vi "ConfigFiles.vi"   [LabVIEW 2016]
uses:
  <vilib>/Utility/config.llb/Read Key (String).vi
  Robot Global Data.vi
  <vilib>/Utility/config.llb/NI_LVConfig.lvlib
types:
  T1 = cluster{" Proportional Gain":dbl, "Integral Time":dbl, "Derivative Time":dbl}
  T2 = typedef "NI_LVConfig.lvlib/Config Data RefNum.ctl" = refnum<k1>
  T3 = cluster{"InchesBack":dbl, "Degrees":dbl, "InchesBack2":dbl, "Degrees2":dbl, "InchesBack3":dbl, "Degrees3":dbl}
  T4 = cluster{"InchesBack":dbl, "Degrees":dbl, "InchesBack2":dbl, "Degrees2":dbl, "InchesBack3":dbl}
  T5 = cluster{"InchesForward":dbl, "Degrees":dbl, "InchesForward2":dbl}
  T6 = cluster{"InchesBack":dbl, "Degrees":dbl, "InchesBack2":dbl}
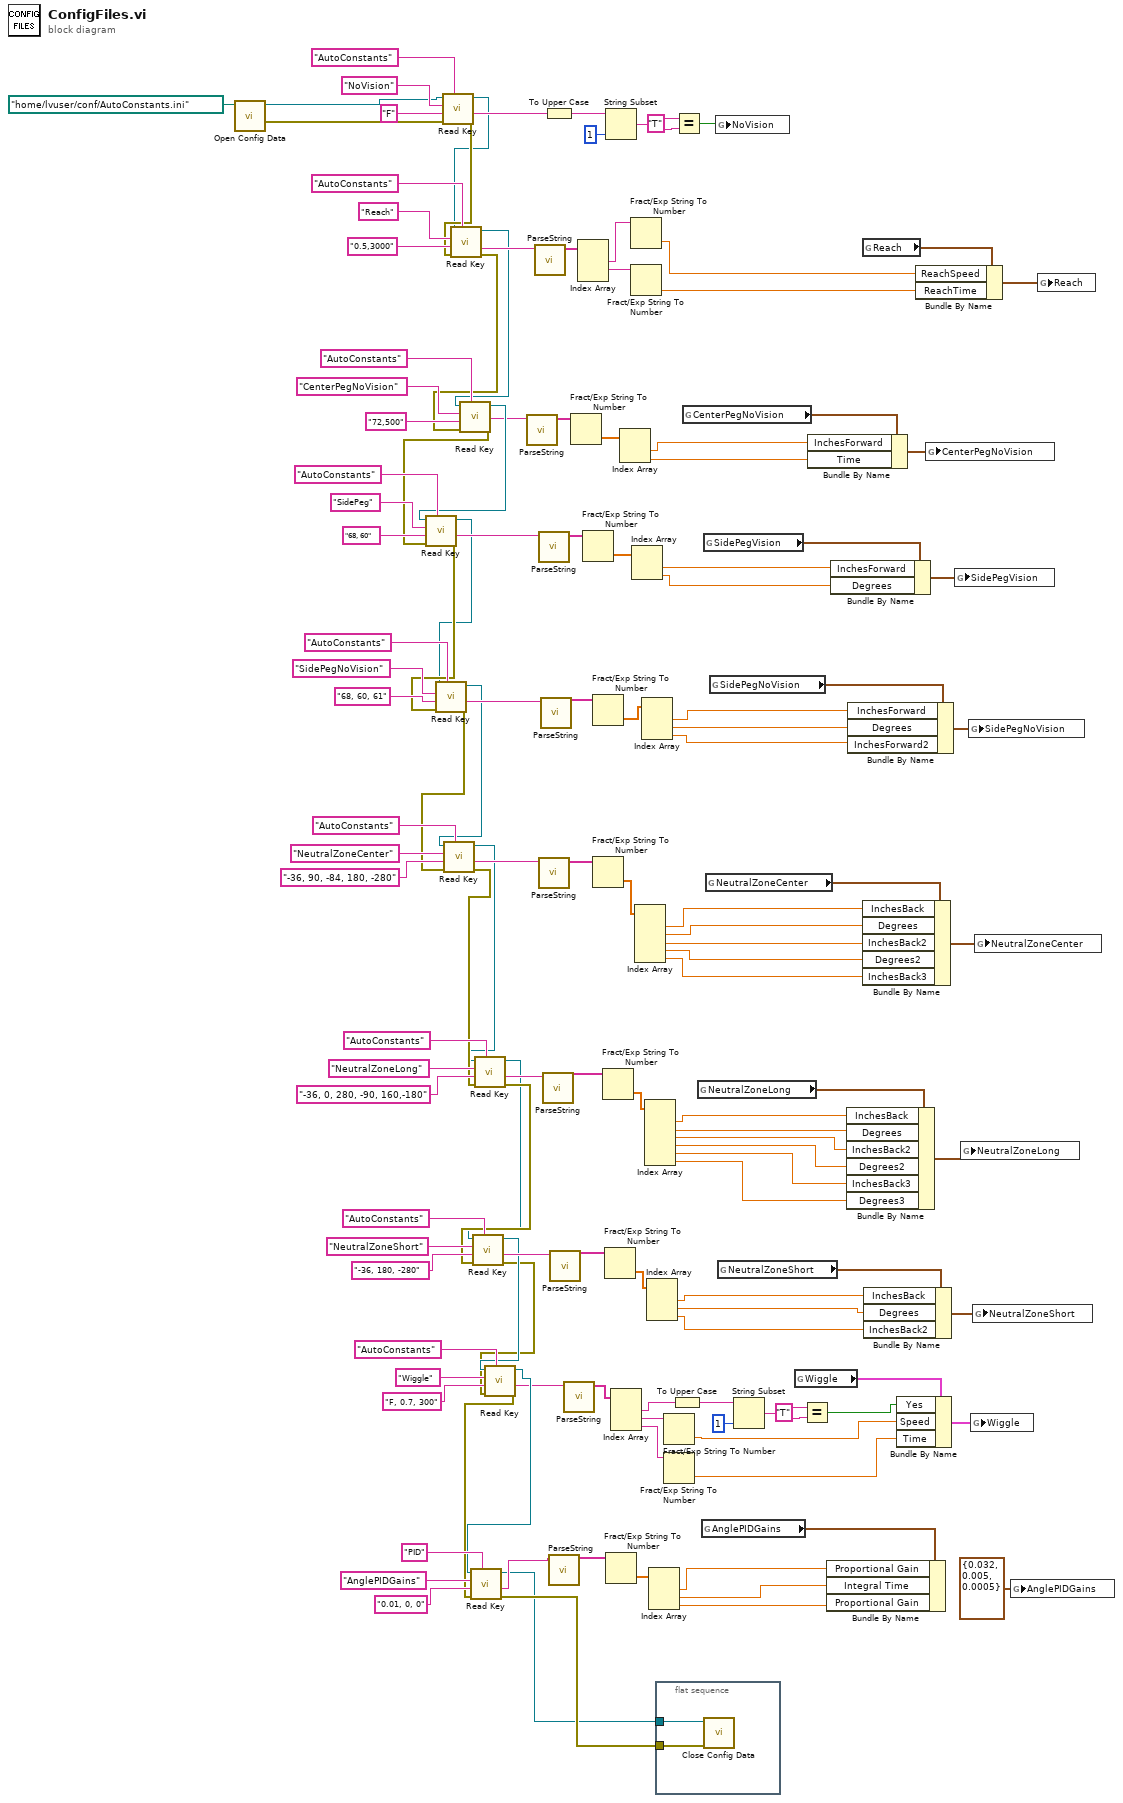
[diagram p0: block diagram]
diagram:
  n1 = call <vilib>:"Open Config Data.vi"("configuration file path"=path "/home/lvuser/conf/AutoConstants.ini") -> ("error out"=w63:errorcluster, "refnum"=w56:T2)  [unwired: 8 in, 1 out]
  n2 = call-poly <vilib>:"Read Key.vi"("section"="AutoConstants", "error in (no error)"=w63, "default value"="F", "key"="NoVision", "refnum"=w56) -> ("error out"=w62:errorcluster, "value"=w126:string, "refnum out"=w55:T2)  [unwired: 3 in, 1 out]
  n3 = call-poly <vilib>:"Read Key.vi"("section"="AutoConstants", "error in (no error)"=w62, "default value"="0.5,3000", "key"="Reach", "refnum"=w55) -> ("error out"=w33:errorcluster, "value"=w66:string, "refnum out"=w32:T2)  [unwired: 3 in, 1 out]
  n4 = call-poly <vilib>:"Read Key.vi"("section"="AutoConstants", "error in (no error)"=w33, "default value"="72,500", "key"="CenterPegNoVision", "refnum"=w32) -> ("error out"=w30:errorcluster, "value"=w27:string, "refnum out"=w31:T2)  [unwired: 3 in, 1 out]
  n5 = call-poly <vilib>:"Read Key.vi"("section"="AutoConstants", "error in (no error)"=w30, "default value"="68, 60", "key"="SidePeg", "refnum"=w31) -> ("error out"=w61:errorcluster, "value"=w68:string, "refnum out"=w54:T2)  [unwired: 3 in, 1 out]
  n6 = call-poly <vilib>:"Read Key.vi"("section"="AutoConstants", "error in (no error)"=w61, "default value"="68, 60, 61", "key"="SidePegNoVision", "refnum"=w54) -> ("error out"=w60:errorcluster, "value"=w70:string, "refnum out"=w53:T2)  [unwired: 3 in, 1 out]
  n7 = call-poly <vilib>:"Read Key.vi"("section"="AutoConstants", "error in (no error)"=w60, "default value"="-36, 90, -84, 180, -280", "key"="NeutralZoneCenter", "refnum"=w53) -> ("error out"=w59:errorcluster, "value"=w72:string, "refnum out"=w52:T2)  [unwired: 3 in, 1 out]
  n8 = call-poly <vilib>:"Read Key.vi"("section"="AutoConstants", "error in (no error)"=w59, "default value"="-36, 0, 280, -90, 160,-180", "key"="NeutralZoneLong", "refnum"=w52) -> ("error out"=w58:errorcluster, "value"=w74:string, "refnum out"=w51:T2)  [unwired: 3 in, 1 out]
  n9 = call-poly <vilib>:"Read Key.vi"("section"="AutoConstants", "error in (no error)"=w58, "default value"="-36, 180, -280", "key"="NeutralZoneShort", "refnum"=w51) -> ("error out"=w18:errorcluster, "value"=w76:string, "refnum out"=w19:T2)  [unwired: 3 in, 1 out]
  n10 = call-poly <vilib>:"Read Key.vi"("section"="AutoConstants", "error in (no error)"=w18, "default value"="F, 0.7, 300", "key"="Wiggle", "refnum"=w19) -> ("error out"=w17:errorcluster, "value"=w15:string, "refnum out"=w16:T2)  [unwired: 3 in, 1 out]
  n11 = call-poly <vilib>:"Read Key.vi"("section"="PID", "error in (no error)"=w17, "default value"="0.01, 0, 0", "key"="AnglePIDGains", "refnum"=w16) -> ("error out"=w57:errorcluster, "value"=w77:string, "refnum out"=w50:T2)  [unwired: 3 in, 1 out]
  n12 = call "ParseString.vi"("String"=w27) -> ("Array"=w29:string[])  [unwired: 10 in]
  n13 = call "ParseString.vi"("String"=w66) -> ("Array"=w65:string[])  [unwired: 10 in]
  n14 = call "ParseString.vi"("String"=w68) -> ("Array"=w67:string[])  [unwired: 10 in]
  n15 = call "ParseString.vi"("String"=w72) -> ("Array"=w71:string[])  [unwired: 10 in]
  n16 = call "ParseString.vi"("String"=w70) -> ("Array"=w69:string[])  [unwired: 10 in]
  n17 = call "ParseString.vi"("String"=w74) -> ("Array"=w73:string[])  [unwired: 10 in]
  n18 = To Upper Case(1:w126) -> (0:w130:string)
  n19 = call "ParseString.vi"("String"=w77) -> ("Array"=w78:string[])  [unwired: 10 in]
  n20 = call "ParseString.vi"("String"=w76) -> ("Array"=w75:string[])  [unwired: 10 in]
  n21 = call "ParseString.vi"("String"=w15) -> ("Array"=w8:string[])  [unwired: 10 in]
  n22 = Fract/Exp String To Number(string=w29) -> (number=w28:dbl[])  [unwired: 3 in, 1 out]
  n23 = Index Array(array=w65) -> (element #1=w138:string, element #2=w137:string)  [unwired: 3 in, 1 out]
  n24 = Fract/Exp String To Number(string=w67) -> (number=w81:dbl[])  [unwired: 3 in, 1 out]
  n25 = Fract/Exp String To Number(string=w69) -> (number=w85:dbl[])  [unwired: 3 in, 1 out]
  n26 = Fract/Exp String To Number(string=w71) -> (number=w92:dbl[])  [unwired: 3 in, 1 out]
  n27 = Fract/Exp String To Number(string=w73) -> (number=w86:dbl[])  [unwired: 3 in, 1 out]
  n28 = Fract/Exp String To Number(string=w75) -> (number=w93:dbl[])  [unwired: 3 in, 1 out]
  n29 = String Subset(string=w130, length (rest)=1 ("length (rest)")) -> (substring=w128:string)  [unwired: 1 in]
  n30 = Fract/Exp String To Number(string=w78) -> (number=w95:dbl[])  [unwired: 3 in, 1 out]
  n31 = Index Array(array=w8) -> (element #1=w7:string, element #2=w13:string, element #3=w6:string)  [unwired: 3 in]
  n32 = Index Array(array=w28) -> (element #1=w25:dbl, element #2=w24:dbl)  [unwired: 2 in]
  n33 = Fract/Exp String To Number(string=w138) -> (number=w133:dbl)  [unwired: 3 in, 1 out]
  n34 = Fract/Exp String To Number(string=w137) -> (number=w134:dbl)  [unwired: 3 in, 1 out]
  n35 = Index Array(array=w81) -> (element #1=w80:dbl, element #2=w79:dbl)  [unwired: 2 in]
  n36 = Index Array(array=w92) -> (element #1=w91:dbl, element #2=w90:dbl, element #3=w89:dbl, element #4=w88:dbl, element #5=w87:dbl)  [unwired: 5 in]
  n37 = Index Array(array=w85) -> (element #1=w84:dbl, element #2=w83:dbl, element #3=w82:dbl)  [unwired: 3 in]
  n38 = Index Array(array=w86) -> (element #1=w48:dbl, element #2=w47:dbl, element #3=w46:dbl, element #4=w45:dbl, element #5=w44:dbl, element #6=w43:dbl)  [unwired: 6 in]
  n39 = Index Array(array=w93) -> (element #1=w42:dbl, element #2=w41:dbl, element #3=w40:dbl)  [unwired: 3 in]
  n40 = Index Array(array=w95) -> (element #1=w39:dbl, element #2=w38:dbl, element #3=w37:dbl)  [unwired: 3 in]
  n41 = flat-sequence {
    tunnel: w57 -> [w142]
    tunnel: w50 -> [w141]
    frame #0 {
      n42 = call <vilib>:"Close Config Data.vi"("error in (no error)"=w142, "refnum"=w141) -> ()  [unwired: 8 in, 2 out]
    }
  }
  n43 = Fract/Exp String To Number(string=w13) -> (number=w2:dbl)  [unwired: 3 in, 1 out]
  n44 = Fract/Exp String To Number(string=w6) -> (number=w1:dbl)  [unwired: 3 in, 1 out]
  n45 = To Upper Case(1:w7) -> (0:w12:string)
  n46 = Equal?(x=w128, y="T") -> (x = y?=w14:bool)
  n47 = global read "Robot Global Data.vi" "CenterPegNoVision"() -> (w26:cluster{"InchesForward":dbl, "Time":dbl})
  n48 = global read "Robot Global Data.vi" "NeutralZoneLong"() -> (w107:T3)
  n49 = global read "Robot Global Data.vi" "AnglePIDGains"() -> (w94:T1)
  n50 = global read "Robot Global Data.vi" "SidePegVision"() -> (w113:cluster{"InchesForward":dbl, "Degrees":dbl})
  n51 = global read "Robot Global Data.vi" "NeutralZoneCenter"() -> (w109:T4)
  n52 = global read "Robot Global Data.vi" "SidePegNoVision"() -> (w110:T5)
  n53 = global write "Robot Global Data.vi" "NoVision"(w14) -> ()
  n54 = global read "Robot Global Data.vi" "NeutralZoneShort"() -> (w104:T6)
  n55 = String Subset(string=w12, length (rest)=1 ("length (rest)")) -> (substring=w10:string)  [unwired: 1 in]
  n56 = global read "Robot Global Data.vi" "Wiggle"() -> (w5:cluster{"Yes":bool, "Speed":dbl, "Time":dbl})
  n57 = Equal?(x=w10, y="T") -> (x = y?=w3:bool)
  n58 = Bundle By Name(cluster=w26, "InchesForward"=w25, "Time"=w24) -> (w23:cluster{"InchesForward":dbl, "Time":dbl})
  n59 = Bundle By Name(cluster=w94, "Proportional Gain"=w39, "Integral Time"=w38, "Proportional Gain"=w37) -> ()  [unwired: 1 out]
  n60 = Bundle By Name(cluster=w113, "InchesForward"=w80, "Degrees"=w79) -> (w112:cluster{"InchesForward":dbl, "Degrees":dbl})
  n61 = Bundle By Name(cluster=w107, "InchesBack"=w48, "Degrees"=w47, "InchesBack2"=w46, "Degrees2"=w45, "InchesBack3"=w44, "Degrees3"=w43) -> (w106:T3)
  n62 = Bundle By Name(cluster=w110, "InchesForward"=w84, "Degrees"=w83, "InchesForward2"=w82) -> (w111:T5)
  n63 = global read "Robot Global Data.vi" "Reach"() -> (w136:cluster{"ReachSpeed":dbl, "ReachTime":dbl})
  n64 = Bundle By Name(cluster=w109, "InchesBack"=w91, "Degrees"=w90, "InchesBack2"=w89, "Degrees2"=w88, "InchesBack3"=w87) -> (w108:T4)
  n65 = Bundle By Name(cluster=w104, "InchesBack"=w42, "Degrees"=w41, "InchesBack2"=w40) -> (w105:T6)
  n66 = Bundle By Name(cluster=w5, "Yes"=w3, "Speed"=w2, "Time"=w1) -> (w4:cluster{"Yes":bool, "Speed":dbl, "Time":dbl})
  n67 = Bundle By Name(cluster=w136, "ReachSpeed"=w133, "ReachTime"=w134) -> (w135:cluster{"ReachSpeed":dbl, "ReachTime":dbl})
  n68 = global write "Robot Global Data.vi" "CenterPegNoVision"(w23) -> ()
  n69 = global write "Robot Global Data.vi" "SidePegVision"(w112) -> ()
  n70 = global write "Robot Global Data.vi" "NeutralZoneLong"(w106) -> ()
  n71 = global write "Robot Global Data.vi" "SidePegNoVision"(w111) -> ()
  n72 = global write "Robot Global Data.vi" "Wiggle"(w4) -> ()
  n73 = global write "Robot Global Data.vi" "NeutralZoneShort"(w105) -> ()
  n74 = global write "Robot Global Data.vi" "NeutralZoneCenter"(w108) -> ()
  n75 = global write "Robot Global Data.vi" "AnglePIDGains"(T1 {" Proportional Gain"=0.032, "Integral Time"=0.005, "Derivative Time"=0.0005} ("AnglePIDGains")) -> ()
  n76 = global write "Robot Global Data.vi" "Reach"(w135) -> ()
